vi "Read Admin Enable.vi"(8 "error in (no error)":errorcluster, 10 "Login PWD":string, 11 "Master in":refnum<class "MASTER.lvclass">) -> (0 "error out":errorcluster, 1 "User Enable":bool, 2 "Admin Enable":bool, 3 "Master out":refnum<class "MASTER.lvclass">)   [LabVIEW 2014, in "Files Library.lvlib" / "Master.lvclass"]
uses:
  MASTER/MASTER.lvclass
  MASTER/MASTER.lvclass/MASTER.ctl
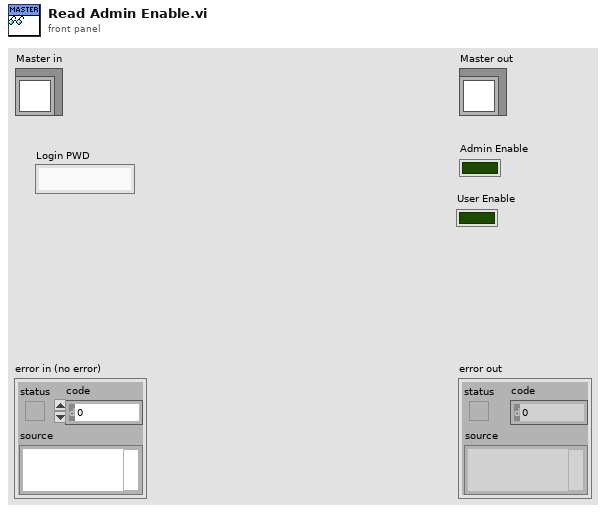
[diagram p1: front panel]
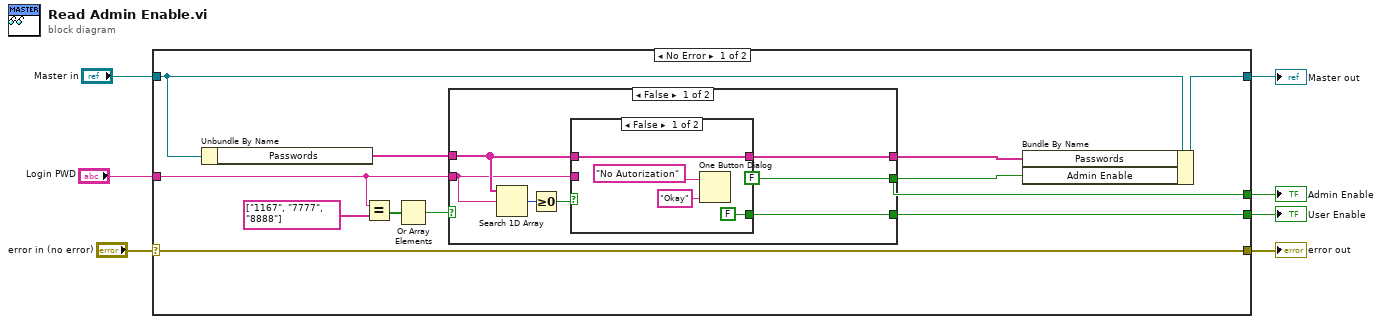
[diagram p0: block diagram]
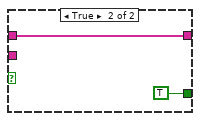
[diagram p2: hidden frame]
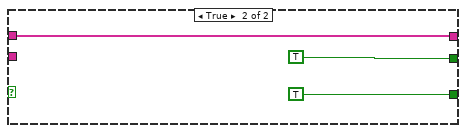
[diagram p3: hidden frame]
diagram:
  n1 = case shown="No Error" "error in (no error)" {
    selector: "error in (no error)" -> [w18 w36]
    tunnel: [w18 w36] -> w3
    tunnel: [w16 w35] -> w5
    tunnel: "Master in" -> [w17 w35]
    tunnel: "Login PWD" -> [w14 _]
    tunnel: [w13 _] -> w4
    tunnel: [w12 _] -> w1
    frame No Error {
      n2 = Unbundle By Name(w17) -> ("Passwords"=w11:string[])
      n3 = Equal?(x=w14, y=string[] ["1167", "7777", "8888"] ("Setting Password.Passwords")) -> (x = y?=w10:bool[])
      n4 = Or Array Elements(Boolean array=w10) -> (logical OR=w8:bool)
      n5 = case shown="False" w8 {
        tunnel: [w25 w34] -> w15
        tunnel: w11 -> [w24 w34]
        tunnel: w14 -> [w21 _]
        tunnel: [FALSE ("Admin Enable") TRUE ("Admin Enable")] -> w13
        tunnel: [w19 TRUE ("User Enable")] -> w12
        frame False {
          n6 = Search 1D Array(1D array=w24, element=w21) -> (index of element=w23:i32)  [unwired: 1 in]
          n7 = Greater Or Equal To 0?(x=w23) -> (x >= 0?=w22:bool)
          n8 = case shown="False" w22 {
            tunnel: [w29 w31] -> w25
            tunnel: w24 -> [w29 w31]
            tunnel: w21 -> [_ _]
            tunnel: [FALSE ("User Enable") TRUE ("User Enable")] -> w19
            frame False {
              n9 = One Button Dialog(message="No Autorization", button name ("OK")="Okay") -> ()  [unwired: 1 out]
            }
            frame True {
            }
          }
        }
        frame True {
        }
      }
      n10 = Bundle By Name(cluster=w17, "Passwords"=w15, "Admin Enable"=w13) -> (w16:refnum<class "MASTER.lvclass">)
    }
    frame Error {
    }
  }
  "error out" <- w3
  "Master out" <- w5
  "Admin Enable" <- w4
  "User Enable" <- w1
